vi "Magna Power.vi"(8 "error in (no error)":errorcluster, 11 "Magna Power in":refnum<class "Magna Power.lvclass">) -> (0 "error out":errorcluster, 3 "Magna Power out":refnum<class "Magna Power.lvclass">)   [LabVIEW 2012, in "Magna Power.lvclass"]
uses:
  Magna Power.lvclass
  Global/GPIB Numbers.vi
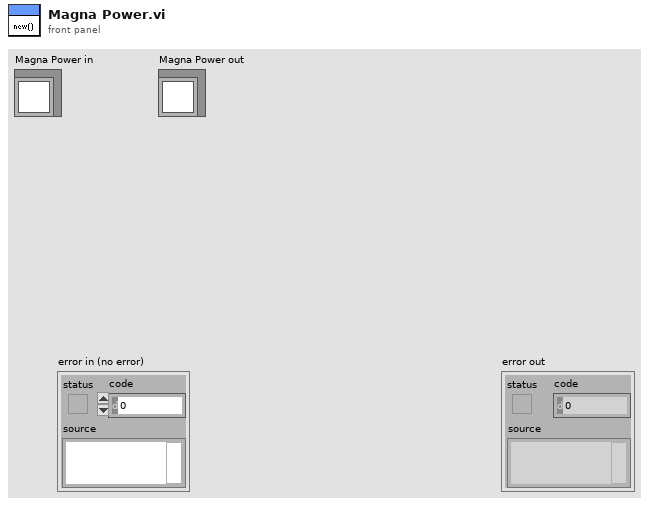
[diagram p1: front panel]
types:
  T1 = cluster{"Name":string, "bus":dbl, "GPIB":dbl, "GPIB as string":string, "byte":i32, "IVI resource name":refnum<k15>, "VISA Resource Name":refnum<visa-resource-name>}
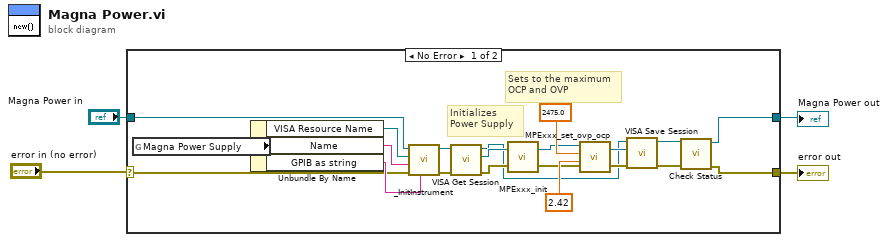
[diagram p0: block diagram]
diagram:
  n1 = case shown="No Error" "error in (no error)" {
    selector: "error in (no error)" -> [w20 w27]
    tunnel: [w6 w27] -> w1
    tunnel: [w5 w26] -> w3
    tunnel: "Magna Power in" -> [w24 w26]
    frame No Error {
      # "Initializes\nPower Supply"
      # "Sets to the maximum\nOCP and OVP"
      n2 = global read "GPIB Numbers.vi" "Magna Power Supply"() -> (w25:T1)
      n3 = Unbundle By Name(w25) -> ("VISA Resource Name"=w23:refnum<visa-resource-name>, "Name"=w21:string, "GPIB as string"=w22:string)
      n4 = call-dynamic "_InitInstrument.vi"("GPIB as string"=w22, "error in (no error)"=w20, "Name"=w21, "VISA Resource Name"=w23, "Instrument in"=w24) -> ("error out"=w18:errorcluster, "Instrument out"=w19:refnum<class "Magna Power.lvclass">)  [unwired: 1 in, 4 out]
      n5 = call-dynamic "VISA Get Session.vi"("error in (no error)"=w18, "Instrument.lvclass in"=w19) -> ("error out"=w13:errorcluster, "VISA Resource Name"=w12:refnum<visa-resource-name>, "Instrument.lvclass out"=w9:refnum<class "Magna Power.lvclass">)  [unwired: 6 in, 1 out]
      n6 = call "MPExxx_init.vi"("error in (no error)"=w13, "VISA session"=w12) -> ("error out"=w14:errorcluster, "dup VISA session"=w15:refnum<visa-resource-name>)
      n7 = call "MPExxx_set_ovp_ocp.vi"("error in (no error)"=w14, "Set OCP"=2.42 ("OCP"), "Set OVP"=2475.0 ("OVP"), "VISA session"=w15) -> ("error out"=w11:errorcluster, "dup VISA session"=w10:refnum<visa-resource-name>)
      n8 = call-dynamic "VISA Save Session.vi"("error in (no error)"=w11, "VISA Resource Name"=w10, "Instrument.lvclass in"=w9) -> ("error out"=w7:errorcluster, "Instrument.lvclass out"=w8:refnum<class "Magna Power.lvclass">)  [unwired: 7 in]
      n9 = call-dynamic "Check Status.vi"("error in (no error)"=w7, "Magna Power in"=w8) -> ("error out"=w6:errorcluster, "Magna Power out"=w5:refnum<class "Magna Power.lvclass">)  [unwired: 6 in, 2 out]
    }
    frame Error {
    }
  }
  "Magna Power out" <- w3
  "error out" <- w1
